vi "Read Write Text File Test.vi"() -> ()   [LabVIEW 2021, in "Test Files.lvlib"]
uses:
  Test Files.lvlib
  <vilib>/addons/_JKI Toolkits/Caraya/classes/Test/Test.lvclass
  <vilib>/addons/_JKI Toolkits/Caraya/classes/Assert/Assert.lvclass
  CustomSortPath.lvlib
  <vilib>/addons/_JKI Toolkits/Caraya/classes/Assert/Assert Equal Value_Variant.vi
  Controls/FileOperation.ctl
panel:
  out "Error Out":errorcluster
  in  "Error In":errorcluster
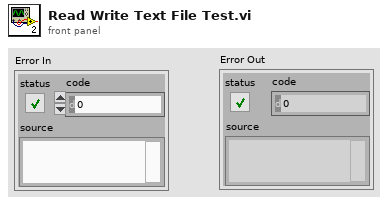
[diagram p1: front panel]
types:
  T1 = typedef "CustomSortPath.lvlib/FileOperation.ctl" = enum16{"Read", "Write"}
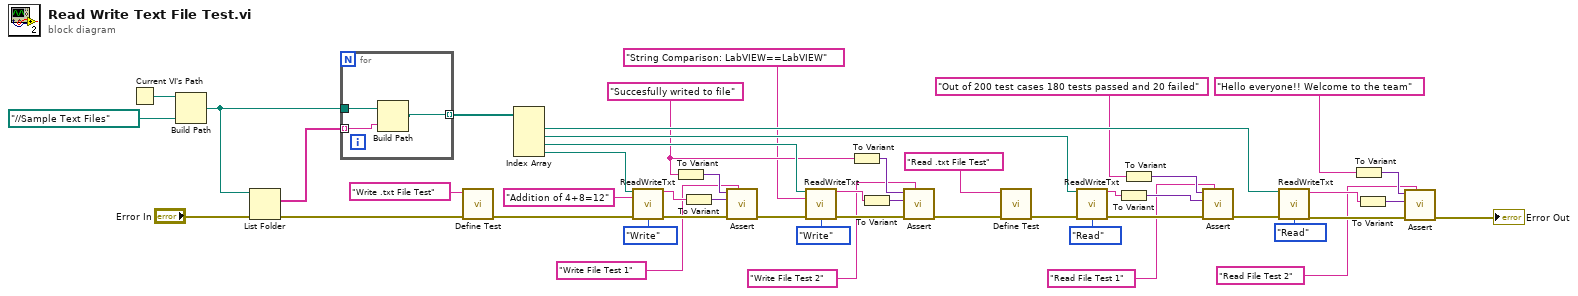
[diagram p0: block diagram]
diagram:
  w13 = "Succesfully writed to file"
  n1 = Current VI's Path() -> (path=w47:path)
  n2 = Build Path(base path=w47, name or relative path=path "../../Sample Text Files") -> (appended path=w42:path)
  n3 = List Folder(path=w42, error in="Error In") -> (filenames=w43:string[], error out=w44:errorcluster)  [unwired: 2 in, 2 out]
  n4 = for {
    tunnel: w43 -> [w50] mode=indexing
    tunnel: w42 -> [w51]
    tunnel: [w49] -> w41 mode=indexing
    n5 = Build Path(base path=w51, name or relative path=w50) -> (appended path=w49:path)
  }
  n6 = call <vilib>:"Define Test.vi"("error in (no error)"=w44, "Label (VI Title)"="Write .txt File Test") -> ("error out"=w15:errorcluster)  [unwired: 8 in, 1 out]
  n7 = Index Array(array=w41) -> (element #1=w40:path, element #2=w33:path, element #3=w24:path, element #4=w22:path)  [unwired: 4 in]
  n8 = call "ReadWriteTxt.vi"("File Path"=w22, "InputString"="Addition of 4+8=12", "error in (no error)"=w15, "FileOperation"=FileOperation."Write") -> ("StringOut"=w19:string, "error out"=w16:errorcluster)  [unwired: 10 in]
  n9 = To Variant(anything=w13) -> (Variant=w21:variant)
  n10 = To Variant(anything=w19) -> (Variant=w20:variant)
  n11 = call-poly <vilib>:"Assert.vi"("Label"="Write File Test 1", "error in (no error)"=w16, "Y"=w20, "X"=w21) -> ("error out"=w17:errorcluster)  [unwired: 6 in, 1 out]
  n12 = call "ReadWriteTxt.vi"("File Path"=w24, "InputString"="String Comparison: LabVIEW==LabVIEW", "error in (no error)"=w17, "FileOperation"=FileOperation."Write") -> ("StringOut"=w11:string, "error out"=w18:errorcluster)  [unwired: 10 in]
  n13 = To Variant(anything=w13) -> (Variant=w12:variant)
  n14 = To Variant(anything=w11) -> (Variant=w10:variant)
  n15 = call-poly <vilib>:"Assert.vi"("Label"="Write File Test 2", "error in (no error)"=w18, "Y"=w10, "X"=w12) -> ("error out"=w9:errorcluster)  [unwired: 6 in, 1 out]
  n16 = call <vilib>:"Define Test.vi"("error in (no error)"=w9, "Label (VI Title)"="Read .txt File Test") -> ("error out"=w8:errorcluster)  [unwired: 8 in, 1 out]
  n17 = call "ReadWriteTxt.vi"("File Path"=w33, "error in (no error)"=w8, "FileOperation"=FileOperation."Read") -> ("StringOut"=w32:string, "error out"=w26:errorcluster)  [unwired: 11 in]
  n18 = To Variant(anything=w32) -> (Variant=w31:variant)
  n19 = To Variant(anything="Out of 200 test cases 180 tests passed and 20 failed") -> (Variant=w29:variant)
  n20 = call-poly <vilib>:"Assert.vi"("Label"="Read File Test 1", "error in (no error)"=w26, "Y"=w31, "X"=w29) -> ("error out"=w28:errorcluster)  [unwired: 6 in, 1 out]
  n21 = call "ReadWriteTxt.vi"("File Path"=w40, "error in (no error)"=w28, "FileOperation"=FileOperation."Read") -> ("StringOut"=w38:string, "error out"=w27:errorcluster)  [unwired: 11 in]
  n22 = To Variant(anything="Hello everyone!! Welcome to the team") -> (Variant=w35:variant)
  n23 = To Variant(anything=w38) -> (Variant=w37:variant)
  n24 = call-poly <vilib>:"Assert.vi"("Label"="Read File Test 2", "error in (no error)"=w27, "Y"=w37, "X"=w35) -> ("error out"=→"Error Out":errorcluster)  [unwired: 6 in, 1 out]
